vi "doOperation.vi"(8 "error in (no error)":errorcluster, 9 "num2":dbl, 10 "num1":dbl, 11 "Strategy in":refnum<class "Strategy.lvclass">) -> (0 "error out":errorcluster, 3 "Strategy out":refnum<class "Strategy.lvclass">)   [LabVIEW 2017, in "Strategy.lvclass"]
uses:
  Strategy.lvclass
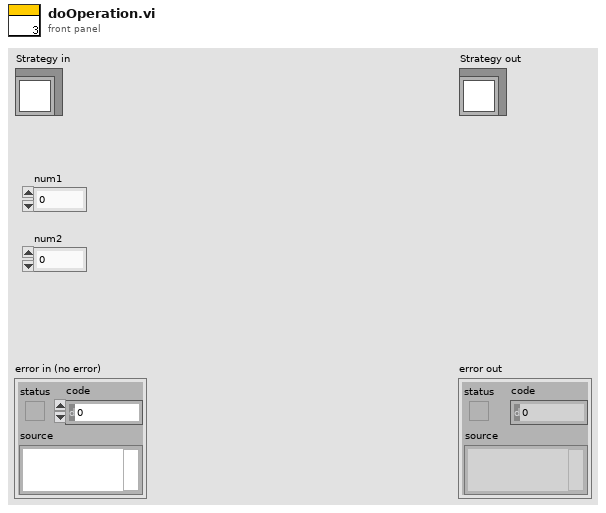
[diagram p1: front panel]
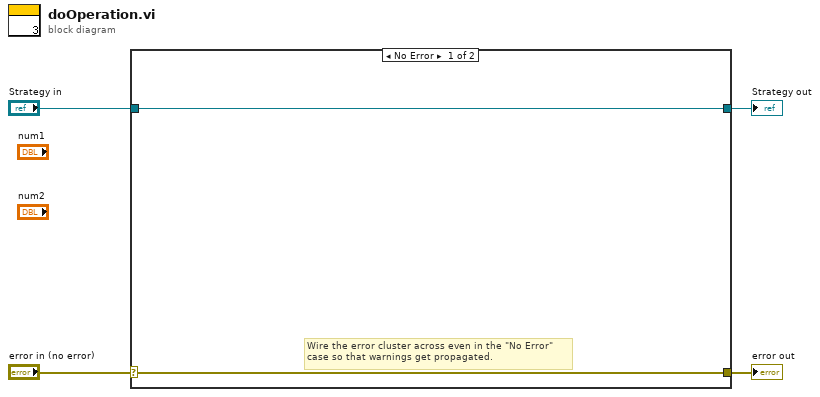
[diagram p0: block diagram]
diagram:
  n1 = case shown="No Error" "error in (no error)" {
    selector: "error in (no error)" -> [w5 w8]
    tunnel: [w5 w8] -> w3
    tunnel: [w6 w7] -> w1
    tunnel: "Strategy in" -> [w6 w7]
    frame No Error {
      # "Wire the error cluster across even in the \"No Error\"\ncase so that warnings get propagated."
    }
    frame Error {
    }
  }
  "error out" <- w3
  "Strategy out" <- w1
